vi "EtherCAT Read by Node U8Array.vi"(7 "dataLen":u32, 8 "error in (no error)":errorcluster, 9 "startAddr":u16, 10 "nodeAddr":u16, 11 "masterHdl in":T1) -> (0 "error out":errorcluster, 2 "data":u8[](array[numeric]), 3 "masterHdl out":T1)   [LabVIEW 2017, in "NI_Robotics_KUKA youBot Host.lvlib"]
uses:
  <vilib>/robotics/KUKA youBot/NI_Robotics_KUKA youBot Host.lvlib
  <vilib>/robotics/KUKA youBot/EtherCAT/LowLevel/Mater Handler.ctl
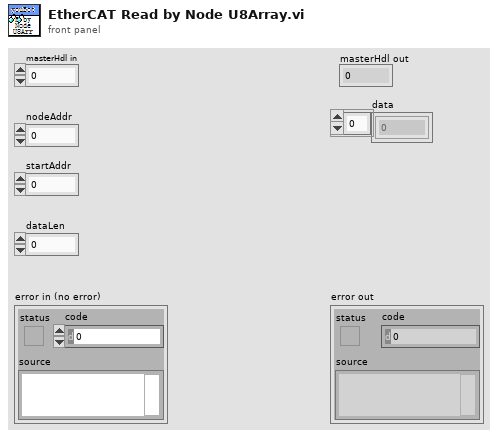
[diagram p1: front panel]
types:
  T1 = typedef "NI_Robotics_KUKA youBot Host.lvlib/Mater Handler.ctl" = i32
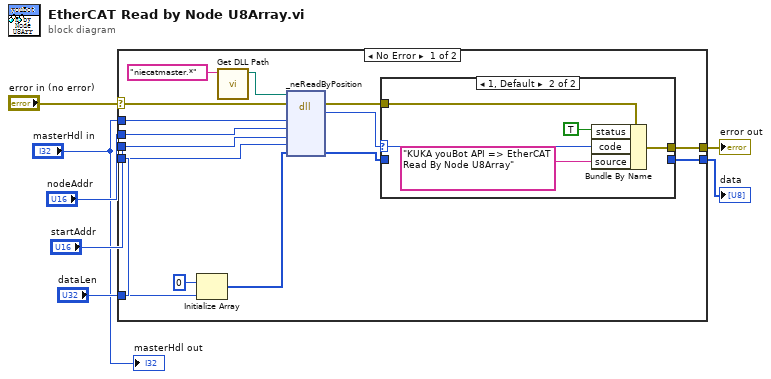
[diagram p0: block diagram]
diagram:
  n1 = case shown="No Error" "error in (no error)" {
    selector: "error in (no error)" -> [w15 w30]
    tunnel: "dataLen" -> [w21 _]
    tunnel: "dataLen" -> [w19 _]
    tunnel: "startAddr" -> [w18 _]
    tunnel: "nodeAddr" -> [w17 _]
    tunnel: "masterHdl in" -> [w16 _]
    tunnel: [w12 w30] -> w3
    tunnel: [w11 _] -> w1
    frame No Error {
      n2 = Initialize Array(u8 0 ("element"), w21) -> (w20:u8[])
      n3 = call <vilib>:"Get DLL Path.vi"("dll name"="niecatmaster.*") -> ("Path"=w8:path)  [unwired: 10 in]
      n4 = dll-call lib="C:/Program Files (x86)/National Instruments/LabVIEW 2012/resource/Framework/Providers/niecatmaster.*" fn="_neReadByPosition"(path in=w8, error in=w15, "masterRef"=w16, "posAddr"=w17, "startAddr"=w18, "dataLen"=w19, "data"=w20) -> (error out=w13:errorcluster, "error"=w14:i32, "data"=w10:u8[])  [unwired: 5 in, 1 out]
      n5 = case shown="1, Default" w14 {
        selector: w14 -> [_ w27]
        tunnel: w13 -> [w24 w26]
        tunnel: [w24 w25] -> w12
        tunnel: [w23 _] -> w11
        tunnel: w10 -> [w23 _]
        frame -2147138411, 0 {
        }
        frame 1, Default {
          n6 = Bundle By Name(cluster=w26, "status"=TRUE, "code"=w27, "source"="KUKA youBot API => EtherCAT Read By Node U8Array") -> (w25:errorcluster)
        }
      }
    }
    frame Error {
    }
  }
  "error out" <- w3
  "data" <- w1
  "masterHdl out" <- "masterHdl in"
